vi "Test Acquisition API.vi"() -> ()   [LabVIEW 2014]
doc: "Acquisition API Tester.\n_____\nBased on Delacor QMH Project Template 4.1.0.59."
uses:
  Acquisition.lvlib
  Settings Editor/Settings Editor.lvlib
panel:
  in  "Settings":bool
  out "error out":errorcluster
  out "Calibrated?":bool
  in  "Calibrate":bool
  out "Waveform Chart":waveform(dbl)[](graph)
  out "Acquiring?":bool
  in  "Stop Acquiring":bool
  out "HW ID":string
  in  "Start Acquiring":bool
  in  "Show Block Diagram":bool
  in  "Stop Module":bool
  in  "Start Module":bool
  in  "Hide Module Panel":bool
  in  "Show Module Panel":bool
  out "Status":string
  out "Module Running?":bool
  # "This VI tests the API for the Module."
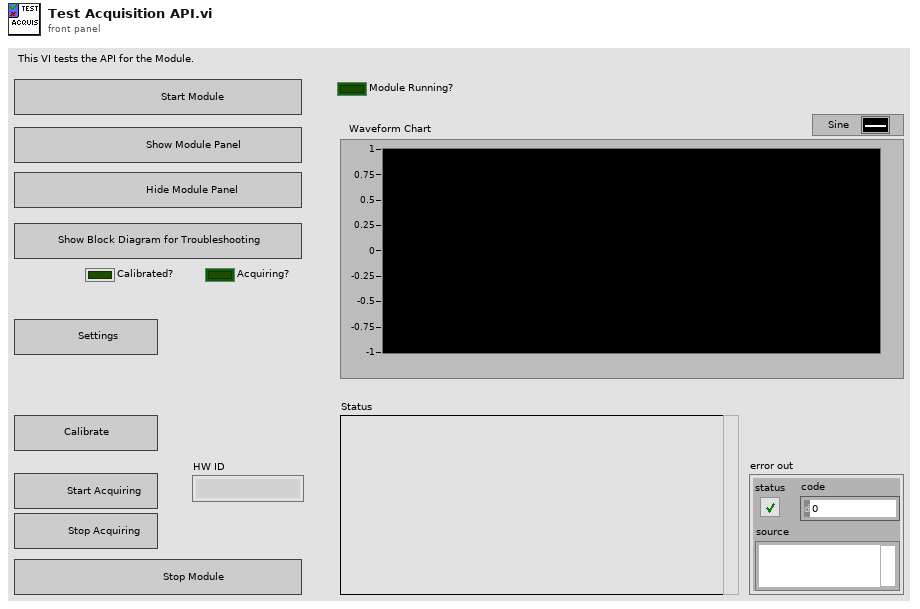
[diagram p1: front panel]
types:
  T1 = typedef "Acquisition.lvlib/Broadcast Events--cluster.ctl" = cluster{"Module Did Init":refnum<user-event>, "Status Updated":refnum<user-event>, "Error Reported":refnum<user-event>, "Module Did Stop":refnum<user-event>, "Update Module Execution Status":refnum<user-event>, "Acquisition Started":refnum<user-event>, "Acquisition Stopped":refnum<user-event>, "Data Updated":refnum<user-event>, "Device Calibrated":refnum<user-event>}
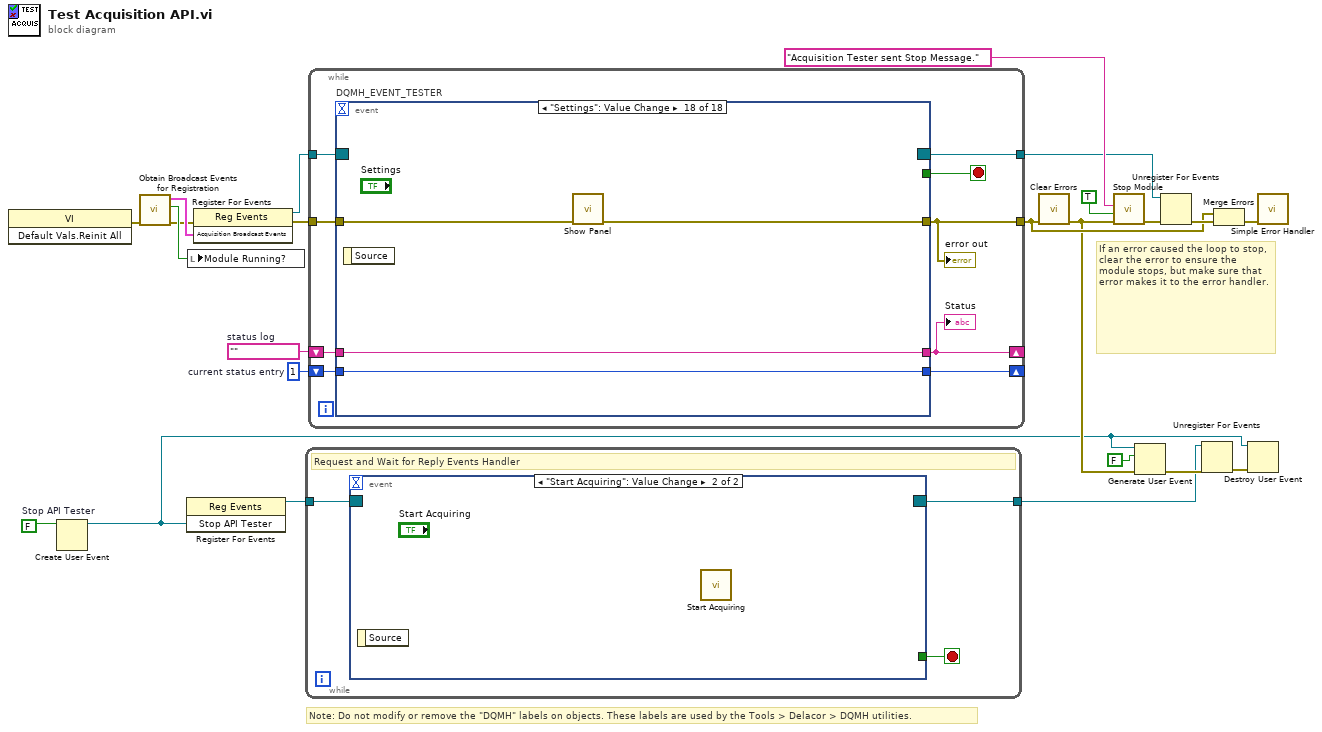
[diagram p0: block diagram]
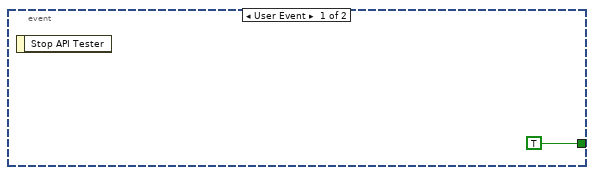
[diagram p2: hidden frame]
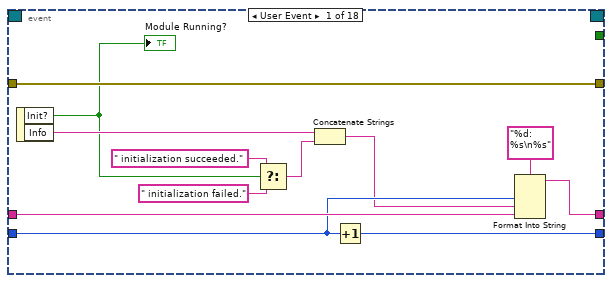
[diagram p3: hidden frame]
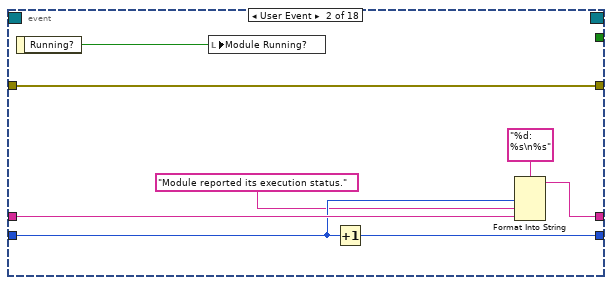
[diagram p4: hidden frame]
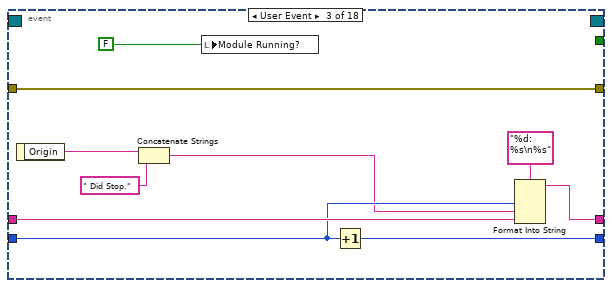
[diagram p5: hidden frame]
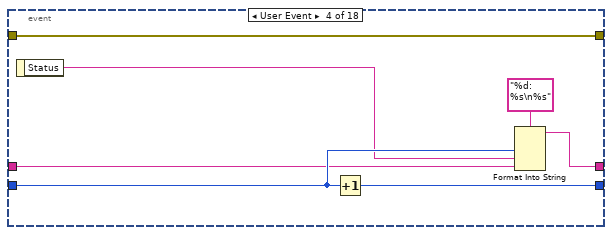
[diagram p6: hidden frame]
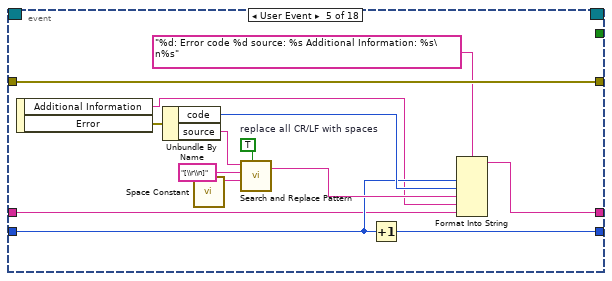
[diagram p7: hidden frame]
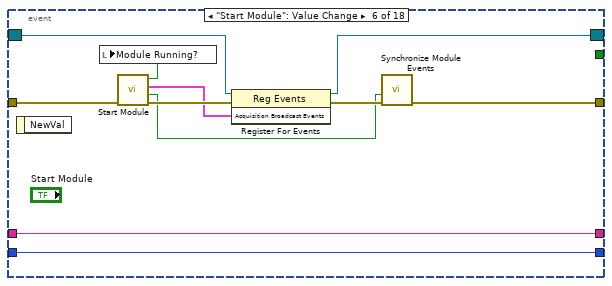
[diagram p8: hidden frame]
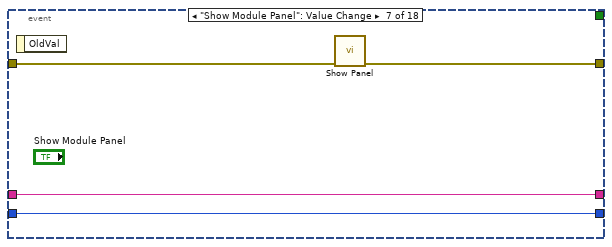
[diagram p9: hidden frame]
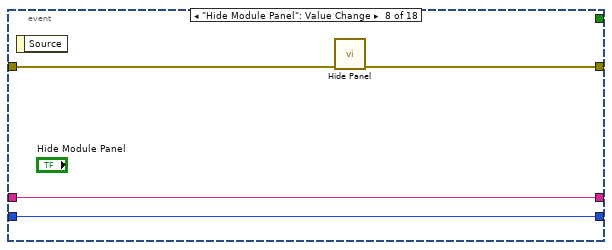
[diagram p10: hidden frame]
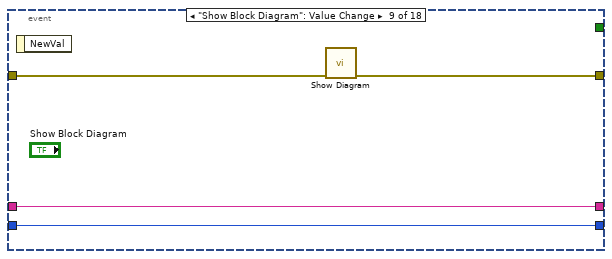
[diagram p11: hidden frame]
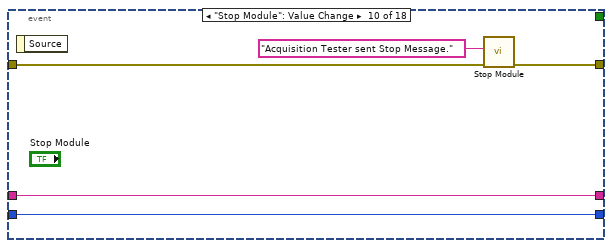
[diagram p12: hidden frame]
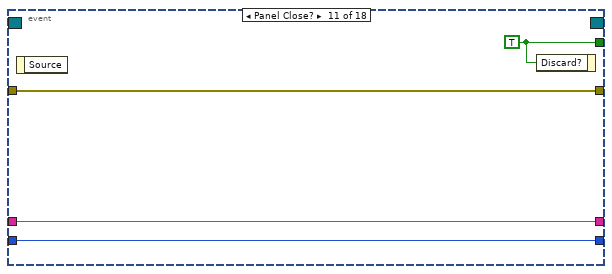
[diagram p13: hidden frame]
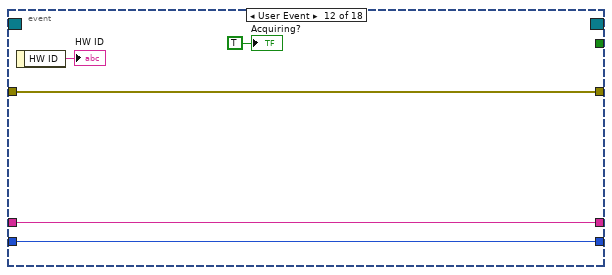
[diagram p14: hidden frame]
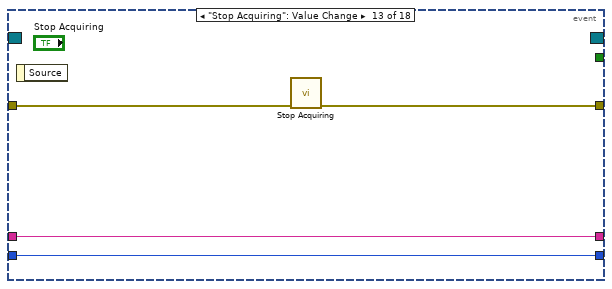
[diagram p15: hidden frame]
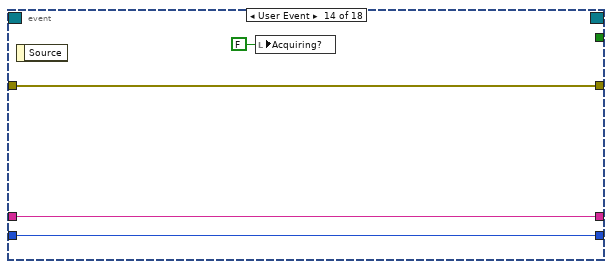
[diagram p16: hidden frame]
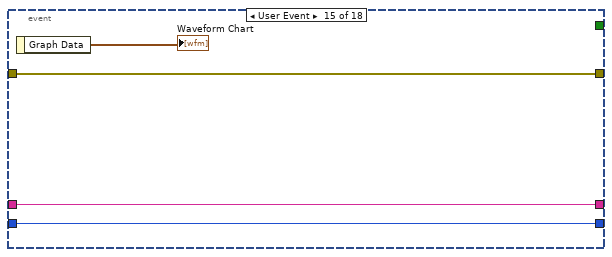
[diagram p17: hidden frame]
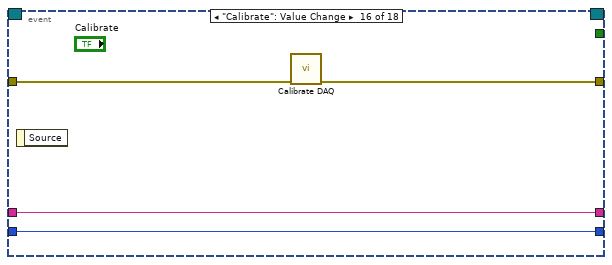
[diagram p18: hidden frame]
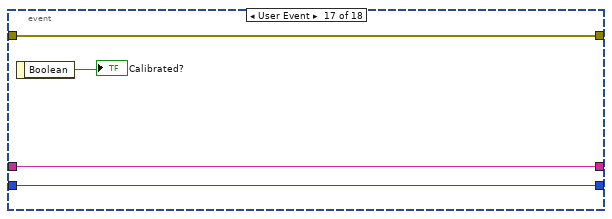
[diagram p19: hidden frame]
diagram:
  w8 = FALSE  # Stop API Tester
  w19 = 1  # current status entry
  w20 = ""  # status log
  # "If an error caused the loop to stop, clear the error to ensure the module stops, but make sure that error makes it to the error handler."
  # "Note: Do not modify or remove the \"DQMH\" labels on objects. These labels are used by the Tools > Delacor > DQMH utilities."
  n1 = invoke on="Invoke Node" class="VI" method="Default Vals.Reinit All"() -> (error out=w10:errorcluster)  [unwired: 3 in, 2 out]
  n2 = Create User Event(user event datatype=w8) -> (user event=w1:refnum<user-event>)  [unwired: 1 in, 1 out]
  n3 = call "Obtain Broadcast Events for Registration.vi"("error in (no error)"=w10) -> ("error out"=w9:errorcluster, "Already running?"=w11:bool, "Acquisition Broadcast Events"=w17:T1)  [unwired: 8 in]
  n4 = register-events(w1) -> (reference out=w7:refnum<event-registration>)  [unwired: 2 in, 1 out]
  n5 = local write "Module Running?"(w11) -> ()
  n6 = register-events(error in=w9, w17) -> (reference out=w16:refnum<event-registration>, error out=w18:errorcluster)  [unwired: 1 in]
  n7 = while {
    tunnel: w7 -> [w26]
    tunnel: [w24] -> w3
    stop <- w25 stop-if-true
    # "Request and Wait for Reply Events Handler"
    n8 = event shown="[1] \"Start Acquiring\": Value Change" {
      selector: w26 -> [_ _]
      dyn-events: [_ _] -> w24
      timeout: _ -> [_ _]
      tunnel: [TRUE _] -> w25
      event User Event {
        n9 = event-data() -> ()  [unwired: 1 in, 1 out]
      }
      event "Start Acquiring": Value Change {
        n10 = event-data() -> ()  [unwired: 1 in, 1 out]
        n11 = call "Start Acquiring.vi"() -> ()  [unwired: 9 in, 3 out]
      }
    }
  }
  n12 = while {
    tunnel: w16 -> [w36]
    tunnel: [w29] -> w12
    shift-right: [w32] -> _
    shift-left: w20 -> [w34]
    shift-right: [w33] -> _
    shift-left: w19 -> [w35]
    tunnel: w18 -> [w31]
    tunnel: [w30] -> w15
    stop <- w28 stop-if-true
    n13 = event "DQMH_EVENT_TESTER" shown="[17] \"Settings\": Value Change" {
      selector: w36 -> [_ _ _ _ _ w92 _ _ _ _ _ _ _ _ _ _ _ _]
      dyn-events: [_ _ _ _ _ w91 _ _ _ _ _ _ _ _ _ _ _ _] -> w30
      timeout: _ -> [_ _ _ _ _ _ _ _ _ _ _ _ _ _ _ _ _ _]
      tunnel: [_ _ _ _ _ _ _ _ _ _ w119 _ _ _ _ _ _ _] -> w28
      tunnel: [w48 w50 w57 w67 w87 w90 w102 w106 w107 w113 w116 w124 w125 w132 w136 w137 w144 w145] -> w29
      tunnel: w35 -> [w45 w54 w64 w70 w77 w95 w100 w104 w108 w114 w117 w122 w126 w130 w134 w138 w142 w147]
      tunnel: w34 -> [w46 w55 w65 w69 w75 w96 w101 w105 w109 w115 w118 w123 w127 w131 w135 w139 w143 w148]
      tunnel: [w43 w52 w62 w71 w78 w96 w101 w105 w109 w115 w118 w123 w127 w131 w135 w139 w143 w148] -> w32
      tunnel: [w44 w53 w63 w73 w76 w95 w100 w104 w108 w114 w117 w122 w126 w130 w134 w138 w142 w147] -> w33
      tunnel: w31 -> [w48 w50 w57 w67 w87 w89 w99 w103 w110 w111 w116 w124 w128 w132 w136 w140 w144 w146]
      event User Event {
        n14 = event-data() -> ("Init?"=w40:bool, "Info"=w42:string)  [unwired: 1 in]
        "Module Running?" <- w40
        n15 = Select(t=" initialization succeeded.", s=w40, f=" initialization failed.") -> (s? t:f=w37:string)
        n16 = Concatenate Strings(w42, w37) -> (w41:string)
        n17 = Increment(x=w45) -> (x+1=w44:i32)
        n18 = Format Into String(format string="%d: %s\n%s", w45, w41, w46) -> (resulting string=w43:string)  [unwired: 2 in, 1 out]
      }
      event User Event {
        n19 = event-data() -> ("Running?"=w49:bool)  [unwired: 1 in]
        n20 = local write "Module Running?"(w49) -> ()
        n21 = Increment(x=w54) -> (x+1=w53:i32)
        n22 = Format Into String(format string="%d: %s\n%s", w54, "Module reported its execution status.", w55) -> (resulting string=w52:string)  [unwired: 2 in, 1 out]
      }
      event User Event {
        n23 = event-data() -> ("Origin"=w61:string)  [unwired: 1 in]
        n24 = Concatenate Strings(w61, " Did Stop.") -> (w60:string)
        n25 = local write "Module Running?"(FALSE ("Module Did Init?")) -> ()
        n26 = Increment(x=w64) -> (x+1=w63:i32)
        n27 = Format Into String(format string="%d: %s\n%s", w64, w60, w65) -> (resulting string=w62:string)  [unwired: 2 in, 1 out]
      }
      event User Event {
        n28 = event-data() -> ("Status"=w68:string)  [unwired: 1 in]
        n29 = Increment(x=w70) -> (x+1=w73:i32)
        n30 = Format Into String(format string="%d: %s\n%s", w70, w68, w69) -> (resulting string=w71:string)  [unwired: 2 in, 1 out]
      }
      event User Event {
        w83 = TRUE  # replace all CR/LF with spaces
        n31 = event-data() -> ("Additional Information"=w74:string, "Error"=w79:errorcluster)  [unwired: 1 in]
        n32 = Unbundle By Name(w79) -> ("code"=w80:i32, "source"=w81:string)
        n33 = call <vilib>:"Space Constant.vi"() -> ("String"=w84:string)
        n34 = call <vilib>:"Search and Replace Pattern.vi"("string"=w81, "regular expression (\"\")"="[\\r\\n]" ("regular expression (\"\")"), "replace string (\"\")"=w84, "replace all? (F)"=w83) -> ("result string"=w82:string)  [unwired: 1 in, 1 out]
        n35 = Increment(x=w77) -> (x+1=w76:i32)
        n36 = Format Into String(format string="%d: Error code %d source: %s Additional Information: %s\n%s", w77, w80, w82, w74, w75) -> (resulting string=w78:string)  [unwired: 2 in, 1 out]
      }
      event "Start Module": Value Change {
        n37 = event-data() -> ()  [unwired: 1 in, 1 out]
        n38 = call "Start Module.vi"("error in (no error)"=w89) -> ("error out"=w97:errorcluster, "Wait for Event Sync?"=w94:bool, "Acquisition Broadcast Events"=w93:T1, "Module Was Already Running?"=w88:bool)  [unwired: 7 in]
        n39 = local write "Module Running?"(w88) -> ()
        n40 = register-events(reference=w92, error in=w97, w93) -> (reference out=w91:refnum<event-registration>, error out=w98:errorcluster)
        n41 = call "Synchronize Module Events.vi"("error in (no error)"=w98, "Wait for Event Sync?"=w94) -> ("error out"=w90:errorcluster)  [unwired: 9 in]
      }
      event "Show Module Panel": Value Change {
        n42 = event-data() -> ()  [unwired: 1 in, 1 out]
        n43 = call "Show Panel.vi"("error in (no error)"=w99) -> ("error out"=w102:errorcluster)  [unwired: 10 in]
      }
      event "Hide Module Panel": Value Change {
        n44 = event-data() -> ()  [unwired: 1 in, 1 out]
        n45 = call "Hide Panel.vi"("error in (no error)"=w103) -> ("error out"=w106:errorcluster)  [unwired: 10 in]
      }
      event "Show Block Diagram": Value Change {
        n46 = event-data() -> ()  [unwired: 1 in, 1 out]
        n47 = call "Show Diagram.vi"("error in (no error)"=w110) -> ("error out"=w107:errorcluster)  [unwired: 10 in]
      }
      event "Stop Module": Value Change {
        n48 = event-data() -> ()  [unwired: 1 in, 1 out]
        n49 = call "Stop Module.vi"("error in (no error)"=w111, "Origin"="Acquisition Tester sent Stop Message.") -> ("error out"=w113:errorcluster)  [unwired: 9 in]
      }
      event Panel Close? {
        w119 = TRUE ("Discard?")
        n50 = event-data() -> ()  [unwired: 1 in, 1 out]
        n51 = event-data ("Event Filter Node")("Discard?"=w119) -> ()  [unwired: 1 in, 1 out]
      }
      event User Event {
        n52 = event-data() -> ("HW ID"=→"HW ID":string)  [unwired: 1 in]
        "Acquiring?" <- TRUE ("Acquiring?")
      }
      event "Stop Acquiring": Value Change {
        n53 = event-data() -> ()  [unwired: 1 in, 1 out]
        n54 = call "Stop Acquiring.vi"("error in (no error)"=w128) -> ("error out"=w125:errorcluster)  [unwired: 10 in]
      }
      event User Event {
        n55 = event-data() -> ()  [unwired: 1 in, 1 out]
        n56 = local write "Acquiring?"(FALSE ("Acquiring?")) -> ()
      }
      event User Event {
        n57 = event-data() -> ("Graph Data"=→"Waveform Chart":waveform(dbl)[])  [unwired: 1 in]
      }
      event "Calibrate": Value Change {
        n58 = event-data() -> ()  [unwired: 1 in, 1 out]
        n59 = call "Calibrate DAQ.vi"("error in (no error)"=w140) -> ("error out"=w137:errorcluster)  [unwired: 10 in]
      }
      event User Event {
        n60 = event-data() -> ("Boolean"=→"Calibrated?":bool)  [unwired: 1 in]
      }
      event "Settings": Value Change {
        n61 = event-data() -> ()  [unwired: 1 in, 1 out]
        n62 = call "Show Panel.vi"("error in (no error)"=w146) -> ("error out"=w145:errorcluster)  [unwired: 10 in]
      }
    }
    "Status" <- w32
    "error out" <- w29
  }
  n63 = call <vilib>:"Clear Errors.vi"("error in (no error)"=w12) -> ("error out"=w6:errorcluster)  [unwired: 5 in, 1 out]
  n64 = call "Stop Module.vi"("error in (no error)"=w6, "Wait for Module to Stop? (F)"=TRUE ("Wait for Module to stop?"), "Origin"="Acquisition Tester sent Stop Message.") -> ("error out"=w22:errorcluster)  [unwired: 8 in]
  n65 = Generate User Event(user event=w1, event data cluster=FALSE ("Stop API Tester"), error in=w6) -> (error out=w4:errorcluster)  [unwired: 1 in, 1 out]
  n66 = Unregister For Events(event registration refnum=w15, error in=w22) -> (error out=w23:errorcluster)
  n67 = Unregister For Events(event registration refnum=w3, error in=w4) -> (error out=w2:errorcluster)
  n68 = Merge Errors(w12, w23) -> (w13:errorcluster)
  n69 = Destroy User Event(user event=w1, error in=w2) -> ()  [unwired: 1 out]
  n70 = call <vilib>:"Simple Error Handler.vi"("error in (no error)"=w13) -> ()  [unwired: 4 in, 5 out]
